vi "Autonomous Independent.vi"() -> ()   [LabVIEW 2016]
doc: "This VI is called when autonomous begins, and will automatically be terminated when autonomous ends. You can carry out timed or sensor driven robot movement independently without needing to return to the caller."
uses:
  <vilib>/Rock Robotics/WPI/Utilities/WPI_GetSetVariantRefNum.vi
  <vilib>/Rock Robotics/Network Tables/NT Read String.vi
  Robot Global Data.vi
  <vilib>/Rock Robotics/Network Tables/NT Write Numeric Array.vi
  <vilib>/Rock Robotics/WPI/RobotDrive/WPI_RobotDriveArcadeDrive_Standard(NoSaturation).vi
panel:
  out "Current Movement, for debugging":T1 {"Y Joystick Value" scale=1.0..-1.0; "X Joystick Value" scale=-1.0..1.0}
  in  "Array of robot movements":T2(array[cluster])=[{"X Joystick Value"=0.39393939393939403, "Y Joystick Value"=0.0, "Delay (sec)"=1.0, "Movement Name"="turn"}, {"X Joystick Value"=-0.3737373737373737, "Y Joystick Value"=0.0, "Delay (sec)"=1.0, "Movement Name"="turn back"}] {"Y Joystick Value" scale=1.0..-1.0; "X Joystick Value" scale=-1.0..1.0}
  # "Be sure to right-click and choose Data Operations>>Make Current Value default if you want to save the array values with the VI"
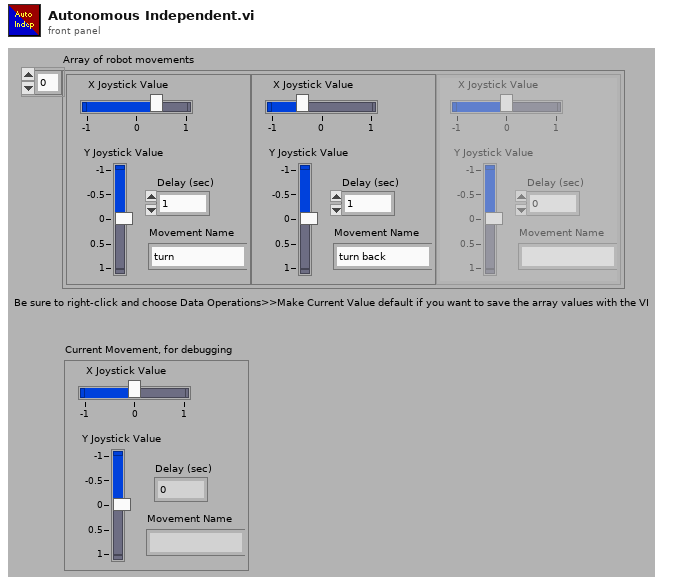
[diagram p1: front panel]
types:
  T1 = cluster{"X Joystick Value":dbl, "Y Joystick Value":dbl, "Delay (sec)":dbl, "Movement Name":string}
  T2 = cluster{"X Joystick Value":dbl, "Y Joystick Value":dbl, "Delay (sec)":dbl, "Movement Name":string}[]
  T3 = typedef "WPI_JoystickDevRef.ctl" = cluster{"Device":T4}
  T4 = typedef "WPI_JoystickDeviceEnum.ctl" = enum16{"USB 0", "USB 1", "USB 2", "USB 3", "USB 4", "USB 5"}
  T5 = typedef "WPI_RobotDriveDevRef.ctl" = cluster{"DevStatus":errorcluster, "Motors[]":T6[], "Square Inputs":bool, "Max Output":dbl}
  T6 = typedef "WPI_MotorControlDeviceRef.ctl" = cluster{"DeviceStatus":errorcluster, "Type":T7, "PWM":cluster{"PWM Channel":T8, "DeadBand":T9}, "CAN":cluster{"Device Number":u8, "SetOutput VI Ref":variant, "GetOutput VI Ref":variant, "Enable VI Ref":variant, "Disable VI Ref":variant, "Data":variant}, "Invert":bool}
  T7 = typedef "WPI_MotorControlType.ctl" = enum16{"PWM", "CAN"}
  T8 = typedef "FPGA_DIOPWMChannel.ctl" = enum8{"PWM 0", "PWM 1", "PWM 2", "PWM 3", "PWM 4", "PWM 5", "PWM 6", "PWM 7", "PWM 8", "PWM 9", "PWM MXP 0", "PWM MXP 1", "PWM MXP 2", "PWM MXP 3", "PWM MXP 4", "PWM MXP 5", "PWM MXP 6", "PWM MXP 7", "PWM MXP 8", "PWM MXP 9", "Invalid"}
  T9 = typedef "WPI_PWMDeadband.ctl" = cluster{"Name":string, "maxPositivePwm":i32, "minPositivePwm":i32, "centerPwm":i32, "maxNegativePwm":i32, "minNegativePwm":i32, "angularRange":u16}
  T10 = enum16{"Move Distance Setup", "Move to Distance", "Move End", "Place Gear Setup", "Place Gear Wait", "Place Gear End", "Angel Move Setup", "Angel Move Wait", "Angel Move End", "End Auto", "WaitForCompletion"}
  T11 = enum16{"Move Distance Setup", "Move to Distance", "Move End", "Place Gear Setup", "Place Gear Wait", "Place Gear End", "Angel Move Setup", "Angel Move Wait", "Angel Move End", "End Auto"}
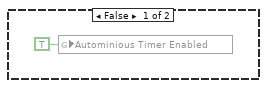
[diagram p6: hidden frame]
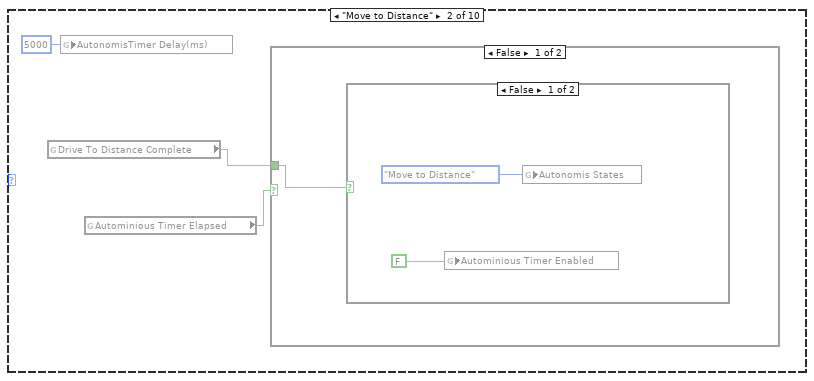
[diagram p7: hidden frame]
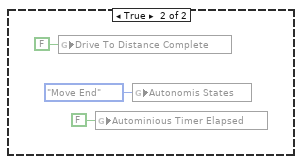
[diagram p8: hidden frame]
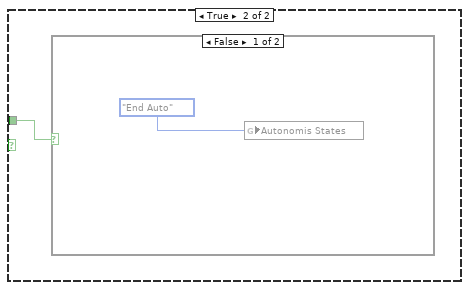
[diagram p9: hidden frame]
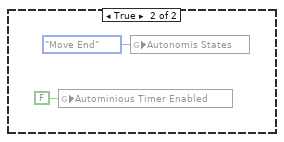
[diagram p10: hidden frame]
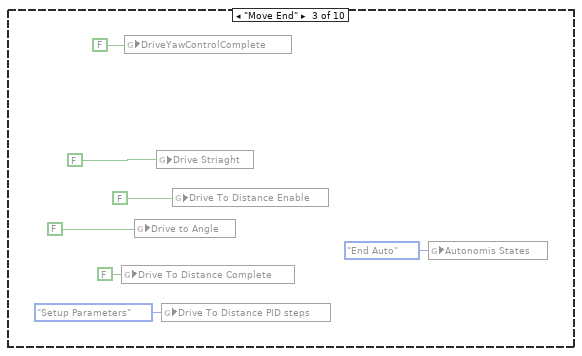
[diagram p11: hidden frame]
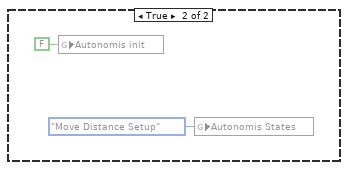
[diagram p19: hidden frame]
diagram:
  (unwired) "This function is run in parallel when the autonomous period begins. It will be terminated automatically when the period ends.\n\nNote that all Driver Station inputs are automatically latched and will not change once auto begins."
  # "initialize values for Move\nenable move to distnace  \nwait for ditance complete\nNext step"
  # "This tells you the autonomous selected\nfrom the dashboard"
  # "Every 20ms, report that we are running autonomous\ncode. Loop will abort the same time as the VI."
  # "This gives you the joystick value\nthat is often the throttle"
  # "This tells you the driver position\nand alliance color"
  n1 = while {
    stop <- FALSE stop-if-true
    n2 = call <vilib>:"WPI_DriverStationReport Robot Code State.vi"("Autonomous"=TRUE) -> ()  [unwired: 10 in, 1 out]
    n3 = Wait (ms)(milliseconds to wait=u32 20) -> ()  [unwired: 1 out]
  }
  n4 = call <vilib>:"WPI_DriverStationGet Alliance Info.vi"() -> ()  [unwired: 12 out]
  n5 = call <vilib>:"WPI_JoystickRefNum Registry Get.vi"("refnum name"="Joystick 0") -> ("JoystickDevRef"=w6:T3)  [unwired: 1 in, 9 out]
  n6 = call <vilib>:"WPI_JoystickGetValues.vi"("JoystickDevRef"=w6) -> ("Axes"=w3:dbl[])  [unwired: 6 in, 4 out]
  n7 = call-poly <vilib>:"NT Read Value.vi"("Name"="Auto Selector") -> ("String"=w1:string)  [unwired: 9 in, 1 out]
  n8 = call-poly <vilib>:"NT Write Value.vi"("Numeric Array"=w3, "Name"="Joystick 0/Axes") -> ()  [unwired: 9 in, 1 out]
  n9 = Index Array(array=w3, index=2) -> ()  [unwired: 1 out]
  n10 = disable-structure shown="Enabled" {
    disable-tunnel: w1 -> [w11 w42]
    frame Disabled {
      # "Use time and/or sensors to control how the robot drives."
      n11 = case shown="\"Alternative 1\"" w11 {
        frame Default {
          # "You can put your main auto here, or you can right-click on the case and make any\nother frame be the default case."
          # "This is the frame that will execute if no selection is made, or if it is not recognized"
        }
        frame "Alternative 1" {
          # "This sample code describes robot movements in an array. You can extend it to control other motors\non your robot. You can also use file I/O to move the data to a text file."
          n12 = call <vilib>:"WPI_RobotDriveRefNum Registry Get.vi"("refnum name"="Left and Right Motors") -> ("RobotDriveDevRef"=w13:T5)  [unwired: 1 in, 9 out]
          n13 = for {
            shift-right: [w21] -> _
            shift-left: w13 -> [w22]
            tunnel: "Array of robot movements" -> [w17] mode=indexing
            n14 = Unbundle By Name(w17) -> ("X Joystick Value"=w20:dbl, "Y Joystick Value"=w19:dbl, "Delay (sec)"=w18:dbl)  [unwired: 1 out]
            n15 = call-poly <vilib>:"WPI_RobotDriveArcadeDrive.vi"("Y axis value"=w19, "X axis value"=w20, "RobotDriveDevRef"=w22) -> ("Motor Values"=w15:dbl[], "RobotDriveDevRef"=w23:T5)  [unwired: 1 in, 6 out]
            n16 = call-poly <vilib>:"NT Write Value.vi"("Numeric Array"=w15, "Name"="RobotDrive Motors") -> ()  [unwired: 9 in, 1 out]
            n17 = call <vilib>:"WPI_RobotDriveDelayAndUpdateSafety.vi"("Delay (s)"=w18, "RobotDriveDevRef"=w23) -> ("RobotDriveDevRef 2"=w21:T5)  [unwired: 8 in, 1 out]
            "Current Movement, for debugging" <- w17
          }
        }
        frame "Alternative 2" {
          w25 = "RobotDrive Motors" ("Name")
          # "This is some simple sample code to drive your robot curving one direction and then the other."
          # "stand still"
          # "other way for 0.5 second"
          # "turn for 1 second"
          n18 = call <vilib>:"WPI_RobotDriveRefNum Registry Get.vi"("refnum name"="Left and Right Motors") -> ("RobotDriveDevRef"=w41:T5)  [unwired: 1 in, 9 out]
          n19 = call-poly <vilib>:"WPI_RobotDriveArcadeDrive.vi"("Y axis value"=0.5 ("X axis value"), "X axis value"=-0.25, "RobotDriveDevRef"=w41) -> ("Motor Values"=w24:dbl[], "RobotDriveDevRef"=w34:T5)  [unwired: 1 in, 6 out]
          n20 = call-poly <vilib>:"NT Write Value.vi"("Numeric Array"=w24, "Name"=w25) -> ()  [unwired: 9 in, 1 out]
          n21 = call <vilib>:"WPI_RobotDriveDelayAndUpdateSafety.vi"("Delay (s)"=1.0, "RobotDriveDevRef"=w34) -> ("RobotDriveDevRef 2"=w35:T5)  [unwired: 8 in, 1 out]
          n22 = call-poly <vilib>:"WPI_RobotDriveArcadeDrive.vi"("Y axis value"=-0.25 ("X axis value"), "X axis value"=0.5, "RobotDriveDevRef"=w35) -> ("Motor Values"=w26:dbl[], "RobotDriveDevRef"=w36:T5)  [unwired: 1 in, 6 out]
          n23 = call-poly <vilib>:"NT Write Value.vi"("Numeric Array"=w26, "Name"=w25) -> ()  [unwired: 9 in, 1 out]
          n24 = call <vilib>:"WPI_RobotDriveDelayAndUpdateSafety.vi"("Delay (s)"=0.5, "RobotDriveDevRef"=w36) -> ("RobotDriveDevRef 2"=w37:T5)  [unwired: 8 in, 1 out]
          n25 = call-poly <vilib>:"WPI_RobotDriveArcadeDrive.vi"("Y axis value"=0.0 ("X axis value"), "X axis value"=0.0, "RobotDriveDevRef"=w37) -> ("Motor Values"=w27:dbl[])  [unwired: 1 in, 7 out]
          n26 = call-poly <vilib>:"NT Write Value.vi"("Numeric Array"=w27, "Name"=w25) -> ()  [unwired: 9 in, 1 out]
        }
        frame "Your Turn" {
        }
      }
    }
    frame Enabled {
      n27 = case shown="\"Right\"" w42 {
        frame "False", Default {
        }
        frame "Do Nothing" {
        }
        frame "Drive Straight" {
          n28 = flat-sequence {
            frame #0 {
              n29 = global write "Robot Global Data.vi" "DriveYawControlComplete"(FALSE ("DriveYawControlRunning")) -> ()
              n30 = global write "Robot Global Data.vi" "Drive To Distance Complete"(FALSE ("Drive To Distance Complete")) -> ()
              n31 = global write "Robot Global Data.vi" "Drive Reset Encoders"(TRUE ("DriveYawControlRunning")) -> ()
              n32 = global write "Robot Global Data.vi" "Drive To Distance Enable"(FALSE ("Drive To Distance Enable")) -> ()
              n33 = global write "Robot Global Data.vi" "Drive to Angle"(FALSE ("Drive To Distance Enable")) -> ()
              n34 = global write "Robot Global Data.vi" "Drive To Distance PID steps"(enum16{"Setup Parameters", "Run PID", "Finish"}."Setup Parameters" ("Drive To Distance PID steps")) -> ()
              n35 = global write "Robot Global Data.vi" "Drive Striaght"(FALSE ("Drive To Distance Enable")) -> ()
              n36 = global write "Robot Global Data.vi" "Drive to Distance setpoint"(115.0 ("Drive to Distance setpoint")) -> ()
              n37 = global write "Robot Global Data.vi" "Nav Reset Yaw"(TRUE ("Drive To Distance Enable")) -> ()
              n38 = Wait (ms)(milliseconds to wait=u32 200) -> ()  [unwired: 1 out]
            }
            frame #1 {
              n39 = global write "Robot Global Data.vi" "Drive To Distance Enable"(TRUE ("Drive To Distance Enable")) -> ()
            }
            frame #2 {
              n40 = while {
                stop <- w55 stop-if-true
                n41 = global read "Robot Global Data.vi" "Drive To Distance Complete"() -> (w55:bool)
                n42 = Wait (ms)(milliseconds to wait=u32 10) -> ()  [unwired: 1 out]
              }
              n43 = global write "Robot Global Data.vi" "Drive Reset Encoders"(FALSE ("DriveYawControlRunning")) -> ()
            }
            frame #3 {
              n44 = global write "Robot Global Data.vi" "Drive To Distance Complete"(FALSE ("Drive To Distance Complete")) -> ()
              n45 = global write "Robot Global Data.vi" "DriveYawControlComplete"(FALSE ("DriveYawControlRunning")) -> ()
              n46 = global write "Robot Global Data.vi" "Drive to Angle"(FALSE ("Drive To Distance Enable")) -> ()
              n47 = global write "Robot Global Data.vi" "Drive Striaght"(FALSE ("Drive To Distance Enable")) -> ()
              n48 = global write "Robot Global Data.vi" "Drive To Distance PID steps"(enum16{"Setup Parameters", "Run PID", "Finish"}."Setup Parameters" ("Drive To Distance PID steps")) -> ()
              n49 = global write "Robot Global Data.vi" "Drive To Distance Enable"(FALSE ("Drive To Distance Enable")) -> ()
            }
            frame #4 {
            }
            frame #5 {
            }
          }
        }
        frame "Left" {
          n50 = flat-sequence {
            frame #0 {
              n51 = global write "Robot Global Data.vi" "DriveYawControlComplete"(FALSE ("DriveYawControlRunning")) -> ()
              n52 = global write "Robot Global Data.vi" "Drive To Distance Complete"(FALSE ("Drive To Distance Complete")) -> ()
              n53 = global write "Robot Global Data.vi" "Drive Reset Encoders"(TRUE ("DriveYawControlRunning")) -> ()
              n54 = global write "Robot Global Data.vi" "Drive To Distance Enable"(FALSE ("Drive To Distance Enable")) -> ()
              n55 = global write "Robot Global Data.vi" "Drive to Angle"(FALSE ("Drive To Distance Enable")) -> ()
              n56 = global write "Robot Global Data.vi" "Drive To Distance PID steps"(enum16{"Setup Parameters", "Run PID", "Finish"}."Setup Parameters" ("Drive To Distance PID steps")) -> ()
              n57 = global write "Robot Global Data.vi" "Drive Striaght"(FALSE ("Drive To Distance Enable")) -> ()
              n58 = global write "Robot Global Data.vi" "Drive to Distance setpoint"(150.0 ("Drive to Distance setpoint")) -> ()
              n59 = global write "Robot Global Data.vi" "Nav Reset Yaw"(TRUE ("Drive To Distance Enable")) -> ()
              n60 = global write "Robot Global Data.vi" "Drive to Distance Direction"(enum16{"Y direction", "X Direction"}."Y direction" ("Drive to Distance Direction")) -> ()
              n61 = Wait (ms)(milliseconds to wait=u32 200) -> ()  [unwired: 1 out]
            }
            frame #1 {
              n62 = global write "Robot Global Data.vi" "Drive To Distance Enable"(TRUE ("Drive To Distance Enable")) -> ()
            }
            frame #2 {
              n63 = while {
                stop <- w76 stop-if-true
                n64 = global read "Robot Global Data.vi" "Drive To Distance Complete"() -> (w76:bool)
                n65 = Wait (ms)(milliseconds to wait=u32 10) -> ()  [unwired: 1 out]
              }
              n66 = global write "Robot Global Data.vi" "Drive Reset Encoders"(FALSE ("DriveYawControlRunning")) -> ()
            }
            frame #3 {
              n67 = global write "Robot Global Data.vi" "Drive To Distance Complete"(FALSE ("Drive To Distance Complete")) -> ()
              n68 = global write "Robot Global Data.vi" "DriveYawControlComplete"(FALSE ("DriveYawControlRunning")) -> ()
              n69 = global write "Robot Global Data.vi" "Drive to Angle"(FALSE ("Drive To Distance Enable")) -> ()
              n70 = global write "Robot Global Data.vi" "Drive Striaght"(FALSE ("Drive To Distance Enable")) -> ()
              n71 = global write "Robot Global Data.vi" "Drive To Distance PID steps"(enum16{"Setup Parameters", "Run PID", "Finish"}."Setup Parameters" ("Drive To Distance PID steps")) -> ()
              n72 = global write "Robot Global Data.vi" "Drive To Distance Enable"(FALSE ("Drive To Distance Enable")) -> ()
            }
            frame #4 {
              n73 = global write "Robot Global Data.vi" "Drive Reset Encoders"(TRUE ("DriveYawControlRunning")) -> ()
              n74 = global write "Robot Global Data.vi" "GearPlace"(TRUE ("GearPlace")) -> ()
            }
            frame #5 {
              n75 = while {
                stop <- w87 stop-if-true
                n76 = global read "Robot Global Data.vi" "GearPlaceComplete"() -> (w87:bool)
                n77 = Wait (ms)(milliseconds to wait=u32 50) -> ()  [unwired: 1 out]
              }
            }
            frame #6 {
              n78 = global write "Robot Global Data.vi" "DriveYawControlComplete"(FALSE ("DriveYawControlRunning")) -> ()
              n79 = global write "Robot Global Data.vi" "Drive To Distance Complete"(FALSE ("Drive To Distance Complete")) -> ()
              n80 = global write "Robot Global Data.vi" "Drive Reset Encoders"(TRUE ("DriveYawControlRunning")) -> ()
              n81 = global write "Robot Global Data.vi" "Drive To Distance Enable"(FALSE ("Drive To Distance Enable")) -> ()
              n82 = global write "Robot Global Data.vi" "Drive to Angle"(FALSE ("Drive To Distance Enable")) -> ()
              n83 = global write "Robot Global Data.vi" "Drive To Distance PID steps"(enum16{"Setup Parameters", "Run PID", "Finish"}."Setup Parameters" ("Drive To Distance PID steps")) -> ()
              n84 = global write "Robot Global Data.vi" "Drive Striaght"(FALSE ("Drive To Distance Enable")) -> ()
              n85 = global write "Robot Global Data.vi" "Drive to Distance Direction"(enum16{"Y direction", "X Direction"}."Y direction" ("Drive to Distance Direction")) -> ()
              n86 = global write "Robot Global Data.vi" "Drive to Distance setpoint"(-12.0 ("Drive to Distance setpoint")) -> ()
              n87 = global write "Robot Global Data.vi" "GearPlace"(FALSE ("GearPlace")) -> ()
              n88 = global write "Robot Global Data.vi" "Nav Reset Yaw"(TRUE ("Drive To Distance Enable")) -> ()
              n89 = Wait (ms)(milliseconds to wait=u32 200) -> ()  [unwired: 1 out]
            }
            frame #7 {
              n90 = global write "Robot Global Data.vi" "Drive To Distance Enable"(TRUE ("Drive To Distance Enable")) -> ()
            }
            frame #8 {
              n91 = while {
                stop <- w102 stop-if-true
                n92 = global read "Robot Global Data.vi" "Drive To Distance Complete"() -> (w102:bool)
                n93 = Wait (ms)(milliseconds to wait=u32 50) -> ()  [unwired: 1 out]
              }
              n94 = global write "Robot Global Data.vi" "Drive Reset Encoders"(FALSE ("DriveYawControlRunning")) -> ()
            }
            frame #9 {
              n95 = global write "Robot Global Data.vi" "Drive To Distance Complete"(FALSE ("Drive To Distance Complete")) -> ()
              n96 = global write "Robot Global Data.vi" "DriveYawControlComplete"(FALSE ("DriveYawControlRunning")) -> ()
              n97 = global write "Robot Global Data.vi" "Drive to Angle"(FALSE ("Drive To Distance Enable")) -> ()
              n98 = global write "Robot Global Data.vi" "Drive Striaght"(FALSE ("Drive To Distance Enable")) -> ()
              n99 = global write "Robot Global Data.vi" "Drive To Distance PID steps"(enum16{"Setup Parameters", "Run PID", "Finish"}."Setup Parameters" ("Drive To Distance PID steps")) -> ()
              n100 = global write "Robot Global Data.vi" "Drive To Distance Enable"(FALSE ("Drive To Distance Enable")) -> ()
            }
            frame #10 {
              n101 = global write "Robot Global Data.vi" "GearPlace"(FALSE ("GearPlace")) -> ()
            }
            frame #11 {
              n102 = disable-structure shown="Disabled" {
                frame Disabled {
                  n103 = global write "Robot Global Data.vi" "DriveYawControlComplete"(FALSE ("DriveYawControlRunning")) -> ()
                  n104 = global write "Robot Global Data.vi" "Drive To Distance Complete"(FALSE ("Drive To Distance Complete")) -> ()
                  n105 = global write "Robot Global Data.vi" "Drive Reset Encoders"(TRUE ("DriveYawControlRunning")) -> ()
                  n106 = global write "Robot Global Data.vi" "Drive To Distance Enable"(FALSE ("Drive To Distance Enable")) -> ()
                  n107 = global write "Robot Global Data.vi" "Drive to Angle"(FALSE ("Drive To Distance Enable")) -> ()
                  n108 = global write "Robot Global Data.vi" "Drive To Distance PID steps"(enum16{"Setup Parameters", "Run PID", "Finish"}."Setup Parameters" ("Drive To Distance PID steps")) -> ()
                  n109 = global write "Robot Global Data.vi" "Drive Striaght"(FALSE ("Drive To Distance Enable")) -> ()
                  n110 = global write "Robot Global Data.vi" "Drive to Distance setpoint"(24.0 ("Drive to Distance setpoint")) -> ()
                  n111 = global write "Robot Global Data.vi" "Gear Holder Open"(FALSE ("Gear Holder Open")) -> ()
                  n112 = global write "Robot Global Data.vi" "Nav Reset Yaw"(TRUE ("Drive To Distance Enable")) -> ()
                  n113 = global write "Robot Global Data.vi" "Drive to Distance Direction"(enum16{"Y direction", "X Direction"}."X Direction" ("Drive to Distance Direction")) -> ()
                  n114 = Wait (ms)(milliseconds to wait=u32 200) -> ()  [unwired: 1 out]
                }
                frame Enabled {
                }
              }
            }
            frame #12 {
              n115 = disable-structure shown="Disabled" {
                frame Disabled {
                  n116 = global write "Robot Global Data.vi" "Drive To Distance Enable"(TRUE ("Drive To Distance Enable")) -> ()
                }
                frame Enabled {
                }
              }
            }
            frame #13 {
              n117 = disable-structure shown="Disabled" {
                frame Disabled {
                  n118 = while {
                    stop <- w125 stop-if-true
                    n119 = global read "Robot Global Data.vi" "Drive To Distance Complete"() -> (w125:bool)
                    n120 = Wait (ms)(milliseconds to wait=u32 10) -> ()  [unwired: 1 out]
                  }
                  n121 = global write "Robot Global Data.vi" "Drive Reset Encoders"(FALSE ("DriveYawControlRunning")) -> ()
                }
                frame Enabled {
                }
              }
            }
            frame #14 {
              n122 = disable-structure shown="Disabled" {
                frame Disabled {
                  n123 = global write "Robot Global Data.vi" "Drive To Distance Complete"(FALSE ("Drive To Distance Complete")) -> ()
                  n124 = global write "Robot Global Data.vi" "DriveYawControlComplete"(FALSE ("DriveYawControlRunning")) -> ()
                  n125 = global write "Robot Global Data.vi" "Drive to Angle"(FALSE ("Drive To Distance Enable")) -> ()
                  n126 = global write "Robot Global Data.vi" "Drive Striaght"(FALSE ("Drive To Distance Enable")) -> ()
                  n127 = global write "Robot Global Data.vi" "Drive To Distance PID steps"(enum16{"Setup Parameters", "Run PID", "Finish"}."Setup Parameters" ("Drive To Distance PID steps")) -> ()
                  n128 = global write "Robot Global Data.vi" "Drive To Distance Enable"(FALSE ("Drive To Distance Enable")) -> ()
                }
                frame Enabled {
                }
              }
            }
          }
        }
        frame "Center" {
          n129 = flat-sequence {
            frame #0 {
              n130 = global write "Robot Global Data.vi" "DriveYawControlComplete"(FALSE ("DriveYawControlRunning")) -> ()
              n131 = global write "Robot Global Data.vi" "Drive To Distance Complete"(FALSE ("Drive To Distance Complete")) -> ()
              n132 = global write "Robot Global Data.vi" "Drive Reset Encoders"(TRUE ("DriveYawControlRunning")) -> ()
              n133 = global write "Robot Global Data.vi" "Drive To Distance Enable"(FALSE ("Drive To Distance Enable")) -> ()
              n134 = global write "Robot Global Data.vi" "Drive to Angle"(FALSE ("Drive To Distance Enable")) -> ()
              n135 = global write "Robot Global Data.vi" "Drive To Distance PID steps"(enum16{"Setup Parameters", "Run PID", "Finish"}."Setup Parameters" ("Drive To Distance PID steps")) -> ()
              n136 = global write "Robot Global Data.vi" "Drive Striaght"(FALSE ("Drive To Distance Enable")) -> ()
              n137 = global write "Robot Global Data.vi" "Drive to Distance setpoint"(100.0 ("Drive to Distance setpoint")) -> ()
              n138 = global write "Robot Global Data.vi" "Nav Reset Yaw"(TRUE ("Drive To Distance Enable")) -> ()
              n139 = global write "Robot Global Data.vi" "Drive to Distance Direction"(enum16{"Y direction", "X Direction"}."Y direction" ("Drive to Distance Direction")) -> ()
              n140 = Wait (ms)(milliseconds to wait=u32 400) -> ()  [unwired: 1 out]
            }
            frame #1 {
              n141 = global write "Robot Global Data.vi" "Drive To Distance Enable"(TRUE ("Drive To Distance Enable")) -> ()
            }
            frame #2 {
              n142 = while {
                stop <- w146 stop-if-true
                n143 = global read "Robot Global Data.vi" "Drive To Distance Complete"() -> (w146:bool)
                n144 = Wait (ms)(milliseconds to wait=u32 10) -> ()  [unwired: 1 out]
              }
              n145 = global write "Robot Global Data.vi" "Drive Reset Encoders"(FALSE ("DriveYawControlRunning")) -> ()
            }
            frame #3 {
              n146 = global write "Robot Global Data.vi" "Drive To Distance Complete"(FALSE ("Drive To Distance Complete")) -> ()
              n147 = global write "Robot Global Data.vi" "DriveYawControlComplete"(FALSE ("DriveYawControlRunning")) -> ()
              n148 = global write "Robot Global Data.vi" "Drive to Angle"(FALSE ("Drive To Distance Enable")) -> ()
              n149 = global write "Robot Global Data.vi" "Drive Striaght"(FALSE ("Drive To Distance Enable")) -> ()
              n150 = global write "Robot Global Data.vi" "Drive To Distance PID steps"(enum16{"Setup Parameters", "Run PID", "Finish"}."Setup Parameters" ("Drive To Distance PID steps")) -> ()
              n151 = global write "Robot Global Data.vi" "Drive To Distance Enable"(FALSE ("Drive To Distance Enable")) -> ()
            }
            frame #4 {
              n152 = global write "Robot Global Data.vi" "Drive Reset Encoders"(TRUE ("DriveYawControlRunning")) -> ()
              n153 = global write "Robot Global Data.vi" "GearPlace"(TRUE ("GearPlace")) -> ()
              n154 = Wait (ms)(milliseconds to wait=u32 10) -> ()  [unwired: 1 out]
            }
            frame #5 {
              n155 = while {
                stop <- w157 stop-if-true
                n156 = global read "Robot Global Data.vi" "GearPlaceComplete"() -> (w157:bool)
                n157 = Wait (ms)(milliseconds to wait=u32 50) -> ()  [unwired: 1 out]
              }
            }
            frame #6 {
              n158 = global write "Robot Global Data.vi" "DriveYawControlComplete"(FALSE ("DriveYawControlRunning")) -> ()
              n159 = global write "Robot Global Data.vi" "Drive To Distance Complete"(FALSE ("Drive To Distance Complete")) -> ()
              n160 = global write "Robot Global Data.vi" "Drive Reset Encoders"(TRUE ("DriveYawControlRunning")) -> ()
              n161 = global write "Robot Global Data.vi" "Drive To Distance Enable"(FALSE ("Drive To Distance Enable")) -> ()
              n162 = global write "Robot Global Data.vi" "Drive to Angle"(FALSE ("Drive To Distance Enable")) -> ()
              n163 = global write "Robot Global Data.vi" "Drive To Distance PID steps"(enum16{"Setup Parameters", "Run PID", "Finish"}."Setup Parameters" ("Drive To Distance PID steps")) -> ()
              n164 = global write "Robot Global Data.vi" "Drive Striaght"(FALSE ("Drive To Distance Enable")) -> ()
              n165 = global write "Robot Global Data.vi" "Drive to Distance Direction"(enum16{"Y direction", "X Direction"}."Y direction" ("Drive to Distance Direction")) -> ()
              n166 = global write "Robot Global Data.vi" "Drive to Distance setpoint"(-12.0 ("Drive to Distance setpoint")) -> ()
              n167 = global write "Robot Global Data.vi" "Nav Reset Yaw"(TRUE ("Drive To Distance Enable")) -> ()
              n168 = global write "Robot Global Data.vi" "GearPlace"(FALSE ("GearPlace")) -> ()
              n169 = Wait (ms)(milliseconds to wait=u32 200) -> ()  [unwired: 1 out]
            }
            frame #7 {
              n170 = global write "Robot Global Data.vi" "Drive To Distance Enable"(TRUE ("Drive To Distance Enable")) -> ()
            }
            frame #8 {
              n171 = while {
                stop <- w173 stop-if-true
                n172 = global read "Robot Global Data.vi" "Drive To Distance Complete"() -> (w173:bool)
                n173 = Wait (ms)(milliseconds to wait=u32 50) -> ()  [unwired: 1 out]
              }
              n174 = global write "Robot Global Data.vi" "Drive Reset Encoders"(FALSE ("DriveYawControlRunning")) -> ()
            }
            frame #9 {
              n175 = global write "Robot Global Data.vi" "Drive To Distance Complete"(FALSE ("Drive To Distance Complete")) -> ()
              n176 = global write "Robot Global Data.vi" "DriveYawControlComplete"(FALSE ("DriveYawControlRunning")) -> ()
              n177 = global write "Robot Global Data.vi" "Drive to Angle"(FALSE ("Drive To Distance Enable")) -> ()
              n178 = global write "Robot Global Data.vi" "Drive Striaght"(FALSE ("Drive To Distance Enable")) -> ()
              n179 = global write "Robot Global Data.vi" "Drive To Distance PID steps"(enum16{"Setup Parameters", "Run PID", "Finish"}."Setup Parameters" ("Drive To Distance PID steps")) -> ()
              n180 = global write "Robot Global Data.vi" "Drive To Distance Enable"(FALSE ("Drive To Distance Enable")) -> ()
            }
          }
        }
        frame "Right" {
          n181 = flat-sequence {
            frame #0 {
              n182 = global write "Robot Global Data.vi" "DriveYawControlComplete"(FALSE ("DriveYawControlRunning")) -> ()
              n183 = global write "Robot Global Data.vi" "Drive To Distance Complete"(FALSE ("Drive To Distance Complete")) -> ()
              n184 = global write "Robot Global Data.vi" "Drive Reset Encoders"(TRUE ("DriveYawControlRunning")) -> ()
              n185 = global write "Robot Global Data.vi" "Drive To Distance Enable"(FALSE ("Drive To Distance Enable")) -> ()
              n186 = global write "Robot Global Data.vi" "Drive to Angle"(FALSE ("Drive To Distance Enable")) -> ()
              n187 = global write "Robot Global Data.vi" "Drive To Distance PID steps"(enum16{"Setup Parameters", "Run PID", "Finish"}."Setup Parameters" ("Drive To Distance PID steps")) -> ()
              n188 = global write "Robot Global Data.vi" "Drive Striaght"(FALSE ("Drive To Distance Enable")) -> ()
              n189 = global write "Robot Global Data.vi" "Drive to Distance setpoint"(150.0 ("Drive to Distance setpoint")) -> ()
              n190 = global write "Robot Global Data.vi" "Nav Reset Yaw"(TRUE ("Drive To Distance Enable")) -> ()
              n191 = global write "Robot Global Data.vi" "Drive to Distance Direction"(enum16{"Y direction", "X Direction"}."Y direction" ("Drive to Distance Direction")) -> ()
              n192 = Wait (ms)(milliseconds to wait=u32 400) -> ()  [unwired: 1 out]
            }
            frame #1 {
              n193 = global write "Robot Global Data.vi" "Drive To Distance Enable"(TRUE ("Drive To Distance Enable")) -> ()
            }
            frame #2 {
              n194 = while {
                stop <- w194 stop-if-true
                n195 = global read "Robot Global Data.vi" "Drive To Distance Complete"() -> (w194:bool)
                n196 = Wait (ms)(milliseconds to wait=u32 50) -> ()  [unwired: 1 out]
              }
              n197 = global write "Robot Global Data.vi" "Drive Reset Encoders"(FALSE ("DriveYawControlRunning")) -> ()
            }
            frame #3 {
              n198 = global write "Robot Global Data.vi" "Drive To Distance Complete"(FALSE ("Drive To Distance Complete")) -> ()
              n199 = global write "Robot Global Data.vi" "DriveYawControlComplete"(FALSE ("DriveYawControlRunning")) -> ()
              n200 = global write "Robot Global Data.vi" "Drive to Angle"(FALSE ("Drive To Distance Enable")) -> ()
              n201 = global write "Robot Global Data.vi" "Drive Striaght"(FALSE ("Drive To Distance Enable")) -> ()
              n202 = global write "Robot Global Data.vi" "Drive To Distance PID steps"(enum16{"Setup Parameters", "Run PID", "Finish"}."Setup Parameters" ("Drive To Distance PID steps")) -> ()
              n203 = global write "Robot Global Data.vi" "Drive To Distance Enable"(FALSE ("Drive To Distance Enable")) -> ()
            }
            frame #4 {
              n204 = global write "Robot Global Data.vi" "Drive Reset Encoders"(TRUE ("DriveYawControlRunning")) -> ()
              n205 = global write "Robot Global Data.vi" "GearPlace"(TRUE ("GearPlace")) -> ()
            }
            frame #5 {
              n206 = while {
                stop <- w205 stop-if-true
                n207 = global read "Robot Global Data.vi" "GearPlaseTimerElapsed"() -> (w205:bool)
                n208 = Wait (ms)(milliseconds to wait=u32 50) -> ()  [unwired: 1 out]
              }
            }
            frame #6 {
              n209 = global write "Robot Global Data.vi" "DriveYawControlComplete"(FALSE ("DriveYawControlRunning")) -> ()
              n210 = global write "Robot Global Data.vi" "Drive To Distance Complete"(FALSE ("Drive To Distance Complete")) -> ()
              n211 = global write "Robot Global Data.vi" "Drive Reset Encoders"(TRUE ("DriveYawControlRunning")) -> ()
              n212 = global write "Robot Global Data.vi" "Drive To Distance Enable"(FALSE ("Drive To Distance Enable")) -> ()
              n213 = global write "Robot Global Data.vi" "Drive to Angle"(FALSE ("Drive To Distance Enable")) -> ()
              n214 = global write "Robot Global Data.vi" "Drive To Distance PID steps"(enum16{"Setup Parameters", "Run PID", "Finish"}."Setup Parameters" ("Drive To Distance PID steps")) -> ()
              n215 = global write "Robot Global Data.vi" "Drive Striaght"(FALSE ("Drive To Distance Enable")) -> ()
              n216 = global write "Robot Global Data.vi" "Drive to Distance Direction"(enum16{"Y direction", "X Direction"}."Y direction" ("Drive to Distance Direction")) -> ()
              n217 = global write "Robot Global Data.vi" "Drive to Distance setpoint"(-12.0 ("Drive to Distance setpoint")) -> ()
              n218 = global write "Robot Global Data.vi" "GearPlace"(FALSE ("GearPlace")) -> ()
              n219 = global write "Robot Global Data.vi" "Nav Reset Yaw"(TRUE ("Drive To Distance Enable")) -> ()
              n220 = Wait (ms)(milliseconds to wait=u32 200) -> ()  [unwired: 1 out]
            }
            frame #7 {
              n221 = global write "Robot Global Data.vi" "Drive To Distance Enable"(TRUE ("Drive To Distance Enable")) -> ()
            }
            frame #8 {
              n222 = while {
                stop <- w221 stop-if-true
                n223 = global read "Robot Global Data.vi" "Drive To Distance Complete"() -> (w221:bool)
                n224 = Wait (ms)(milliseconds to wait=u32 50) -> ()  [unwired: 1 out]
              }
              n225 = global write "Robot Global Data.vi" "Drive Reset Encoders"(FALSE ("DriveYawControlRunning")) -> ()
            }
            frame #9 {
              n226 = global write "Robot Global Data.vi" "Drive To Distance Complete"(FALSE ("Drive To Distance Complete")) -> ()
              n227 = global write "Robot Global Data.vi" "DriveYawControlComplete"(FALSE ("DriveYawControlRunning")) -> ()
              n228 = global write "Robot Global Data.vi" "Drive to Angle"(FALSE ("Drive To Distance Enable")) -> ()
              n229 = global write "Robot Global Data.vi" "Drive Striaght"(FALSE ("Drive To Distance Enable")) -> ()
              n230 = global write "Robot Global Data.vi" "Drive To Distance PID steps"(enum16{"Setup Parameters", "Run PID", "Finish"}."Setup Parameters" ("Drive To Distance PID steps")) -> ()
              n231 = global write "Robot Global Data.vi" "Drive To Distance Enable"(FALSE ("Drive To Distance Enable")) -> ()
            }
            frame #10 {
              n232 = disable-structure shown="Disabled" {
                frame Disabled {
                  n233 = global write "Robot Global Data.vi" "DriveYawControlComplete"(FALSE ("DriveYawControlRunning")) -> ()
                  n234 = global write "Robot Global Data.vi" "Drive To Distance Complete"(FALSE ("Drive To Distance Complete")) -> ()
                  n235 = global write "Robot Global Data.vi" "Drive Reset Encoders"(TRUE ("DriveYawControlRunning")) -> ()
                  n236 = global write "Robot Global Data.vi" "Drive To Distance Enable"(FALSE ("Drive To Distance Enable")) -> ()
                  n237 = global write "Robot Global Data.vi" "Drive to Angle"(FALSE ("Drive To Distance Enable")) -> ()
                  n238 = global write "Robot Global Data.vi" "Drive To Distance PID steps"(enum16{"Setup Parameters", "Run PID", "Finish"}."Setup Parameters" ("Drive To Distance PID steps")) -> ()
                  n239 = global write "Robot Global Data.vi" "Drive Striaght"(FALSE ("Drive To Distance Enable")) -> ()
                  n240 = global write "Robot Global Data.vi" "Drive to Distance setpoint"(-24.0 ("Drive to Distance setpoint")) -> ()
                  n241 = global write "Robot Global Data.vi" "Gear Holder Open"(FALSE ("Gear Holder Open")) -> ()
                  n242 = global write "Robot Global Data.vi" "Nav Reset Yaw"(TRUE ("Drive To Distance Enable")) -> ()
                  n243 = global write "Robot Global Data.vi" "Drive to Distance Direction"(enum16{"Y direction", "X Direction"}."X Direction" ("Drive to Distance Direction")) -> ()
                  n244 = Wait (ms)(milliseconds to wait=u32 200) -> ()  [unwired: 1 out]
                }
                frame Enabled {
                }
              }
            }
            frame #11 {
              n245 = disable-structure shown="Disabled" {
                frame Disabled {
                  n246 = global write "Robot Global Data.vi" "Drive To Distance Enable"(TRUE ("Drive To Distance Enable")) -> ()
                }
                frame Enabled {
                }
              }
            }
            frame #12 {
              n247 = disable-structure shown="Disabled" {
                frame Disabled {
                  n248 = while {
                    stop <- w242 stop-if-true
                    n249 = global read "Robot Global Data.vi" "Drive To Distance Complete"() -> (w242:bool)
                    n250 = Wait (ms)(milliseconds to wait=u32 10) -> ()  [unwired: 1 out]
                  }
                  n251 = global write "Robot Global Data.vi" "Drive Reset Encoders"(FALSE ("DriveYawControlRunning")) -> ()
                }
                frame Enabled {
                }
              }
            }
            frame #13 {
              n252 = disable-structure shown="Disabled" {
                frame Disabled {
                  n253 = global write "Robot Global Data.vi" "Drive To Distance Complete"(FALSE ("Drive To Distance Complete")) -> ()
                  n254 = global write "Robot Global Data.vi" "DriveYawControlComplete"(FALSE ("DriveYawControlRunning")) -> ()
                  n255 = global write "Robot Global Data.vi" "Drive to Angle"(FALSE ("Drive To Distance Enable")) -> ()
                  n256 = global write "Robot Global Data.vi" "Drive Striaght"(FALSE ("Drive To Distance Enable")) -> ()
                  n257 = global write "Robot Global Data.vi" "Drive To Distance PID steps"(enum16{"Setup Parameters", "Run PID", "Finish"}."Setup Parameters" ("Drive To Distance PID steps")) -> ()
                  n258 = global write "Robot Global Data.vi" "Drive to Distance Direction"(enum16{"Y direction", "X Direction"}."Y direction" ("Drive to Distance Direction")) -> ()
                  n259 = global write "Robot Global Data.vi" "Drive To Distance Enable"(FALSE ("Drive To Distance Enable")) -> ()
                }
                frame Enabled {
                }
              }
            }
          }
        }
      }
    }
  }
  n260 = disable-structure shown="Disabled" {
    disable-tunnel: w1 -> [w251 _]
    frame Disabled {
      n261 = case shown="\"Right\"" w251 {
        frame "Do Nothing", Default {
        }
        frame "Center" {
        }
        frame "Drive Straight" {
        }
        frame "Left" {
        }
        frame "Right" {
          n262 = global read "Robot Global Data.vi" "Autonomis init"() -> (w252:bool)
          n263 = case shown="False" w252 {
            frame False {
              n264 = global read "Robot Global Data.vi" "Autonomis States"() -> (w253:T10)
              n265 = case shown="\"Move Distance Setup\", Default" w253 {
                frame "Move Distance Setup", Default {
                  n266 = global write "Robot Global Data.vi" "DriveYawControlComplete"(FALSE ("DriveYawControlRunning")) -> ()
                  n267 = global write "Robot Global Data.vi" "Drive To Distance Complete"(FALSE ("Drive To Distance Complete")) -> ()
                  n268 = global write "Robot Global Data.vi" "Drive Reset Encoders"(TRUE ("DriveYawControlRunning")) -> ()
                  n269 = global write "Robot Global Data.vi" "Drive To Distance Enable"(FALSE ("Drive To Distance Enable")) -> ()
                  n270 = global write "Robot Global Data.vi" "Drive to Angle"(FALSE ("Drive To Distance Enable")) -> ()
                  n271 = global write "Robot Global Data.vi" "Drive Striaght"(FALSE ("Drive To Distance Enable")) -> ()
                  n272 = global write "Robot Global Data.vi" "Nav Reset Yaw"(TRUE ("Drive To Distance Enable")) -> ()
                  n273 = global write "Robot Global Data.vi" "Drive to Distance setpoint"(115.0 ("Drive to Distance setpoint")) -> ()
                  n274 = global read "Robot Global Data.vi" "Autominious Timer Elapsed"() -> (w255:bool)
                  n275 = global write "Robot Global Data.vi" "AutonomisTimer Delay(ms)"(u32 200 ("AutonomisTimer Delay(ms)")) -> ()
                  n276 = case shown="True" w255 {
                    frame False {
                      n277 = global write "Robot Global Data.vi" "Autominious Timer Enabled"(TRUE ("Autominious Timer Enabled")) -> ()
                    }
                    frame True {
                      n278 = global write "Robot Global Data.vi" "Drive To Distance Enable"(FALSE ("Drive To Distance Enable")) -> ()
                      n279 = global write "Robot Global Data.vi" "Drive Reset Encoders"(FALSE ("DriveYawControlRunning")) -> ()
                      n280 = global write "Robot Global Data.vi" "Autominious Timer Enabled"(FALSE ("Autominious Timer Enabled")) -> ()
                      n281 = global write "Robot Global Data.vi" "Autonomis States"(T10."Move to Distance" ("Autonomis States")) -> ()
                    }
                  }
                }
                frame "Move to Distance" {
                  n282 = global read "Robot Global Data.vi" "Drive To Distance Complete"() -> (w271:bool)
                  n283 = global write "Robot Global Data.vi" "AutonomisTimer Delay(ms)"(u32 5000 ("AutonomisTimer Delay(ms)")) -> ()
                  n284 = global read "Robot Global Data.vi" "Autominious Timer Elapsed"() -> (w269:bool)
                  n285 = case shown="False" w269 {
                    tunnel: w271 -> [w272 w278]
                    frame False {
                      n286 = case shown="False" w272 {
                        frame False {
                          n287 = global write "Robot Global Data.vi" "Autominious Timer Enabled"(FALSE ("Autominious Timer Enabled")) -> ()
                          n288 = global write "Robot Global Data.vi" "Autonomis States"(T10."Move to Distance" ("Autonomis States")) -> ()
                        }
                        frame True {
                          n289 = global write "Robot Global Data.vi" "Drive To Distance Complete"(FALSE ("Drive To Distance Complete")) -> ()
                          n290 = global write "Robot Global Data.vi" "Autominious Timer Elapsed"(FALSE ("Autominious Timer Elapsed")) -> ()
                          n291 = global write "Robot Global Data.vi" "Autonomis States"(T10."Move End" ("Autonomis States")) -> ()
                        }
                      }
                    }
                    frame True {
                      n292 = case shown="False" w278 {
                        frame False {
                          n293 = global write "Robot Global Data.vi" "Autonomis States"(T10."End Auto" ("Autonomis States")) -> ()
                        }
                        frame True {
                          n294 = global write "Robot Global Data.vi" "Autominious Timer Enabled"(FALSE ("Autominious Timer Enabled")) -> ()
                          n295 = global write "Robot Global Data.vi" "Autonomis States"(T10."Move End" ("Autonomis States")) -> ()
                        }
                      }
                    }
                  }
                }
                frame "Move End" {
                  n296 = global write "Robot Global Data.vi" "Drive To Distance Complete"(FALSE ("Drive To Distance Complete")) -> ()
                  n297 = global write "Robot Global Data.vi" "DriveYawControlComplete"(FALSE ("DriveYawControlRunning")) -> ()
                  n298 = global write "Robot Global Data.vi" "Drive to Angle"(FALSE ("Drive To Distance Enable")) -> ()
                  n299 = global write "Robot Global Data.vi" "Drive Striaght"(FALSE ("Drive To Distance Enable")) -> ()
                  n300 = global write "Robot Global Data.vi" "Drive To Distance PID steps"(enum16{"Setup Parameters", "Run PID", "Finish"}."Setup Parameters" ("Drive To Distance PID steps")) -> ()
                  n301 = global write "Robot Global Data.vi" "Drive To Distance Enable"(FALSE ("Drive To Distance Enable")) -> ()
                  n302 = global write "Robot Global Data.vi" "Autonomis States"(T10."End Auto" ("Autonomis States")) -> ()
                }
                frame "Place Gear Setup" {
                }
                frame "Place Gear Wait" {
                }
                frame "Place Gear End" {
                }
                frame "Angel Move Setup" {
                }
                frame "Angel Move Wait" {
                }
                frame "Angel Move End" {
                }
                frame "End Auto" {
                }
              }
            }
            frame True {
              n303 = global write "Robot Global Data.vi" "Autonomis init"(FALSE ("Autonomis init")) -> ()
              n304 = global write "Robot Global Data.vi" "Autonomis States"(T11."Move Distance Setup" ("Autonomis States")) -> ()
            }
          }
        }
      }
    }
    frame Enabled {
    }
  }
  n305 = disable-structure shown="Disabled" {
    frame Disabled {
      n306 = flat-sequence {
        frame #0 {
          n307 = global write "Robot Global Data.vi" "DriveYawControlComplete"(FALSE ("DriveYawControlRunning")) -> ()
          n308 = global write "Robot Global Data.vi" "Drive To Distance Complete"(FALSE ("Drive To Distance Complete")) -> ()
          n309 = global write "Robot Global Data.vi" "Drive Reset Encoders"(TRUE ("DriveYawControlRunning")) -> ()
          n310 = global write "Robot Global Data.vi" "Drive To Distance Enable"(FALSE ("Drive To Distance Enable")) -> ()
          n311 = global write "Robot Global Data.vi" "Drive to Angle"(FALSE ("Drive To Distance Enable")) -> ()
          n312 = global write "Robot Global Data.vi" "Drive To Distance PID steps"(enum16{"Setup Parameters", "Run PID", "Finish"}."Setup Parameters" ("Drive To Distance PID steps")) -> ()
          n313 = global write "Robot Global Data.vi" "Drive Striaght"(FALSE ("Drive To Distance Enable")) -> ()
          n314 = global write "Robot Global Data.vi" "Drive to Distance setpoint"(75.0 ("Drive to Distance setpoint")) -> ()
          n315 = global write "Robot Global Data.vi" "Nav Reset Yaw"(TRUE ("Drive To Distance Enable")) -> ()
          n316 = Wait (ms)(milliseconds to wait=u32 200) -> ()  [unwired: 1 out]
        }
        frame #1 {
          n317 = global write "Robot Global Data.vi" "Drive To Distance Enable"(TRUE ("Drive To Distance Enable")) -> ()
        }
        frame #2 {
          n318 = while {
            stop <- w303 stop-if-true
            n319 = global read "Robot Global Data.vi" "Drive To Distance Complete"() -> (w303:bool)
            n320 = Wait (ms)(milliseconds to wait=u32 10) -> ()  [unwired: 1 out]
          }
          n321 = global write "Robot Global Data.vi" "Drive Reset Encoders"(FALSE ("DriveYawControlRunning")) -> ()
        }
        frame #3 {
          n322 = global write "Robot Global Data.vi" "Drive To Distance Complete"(FALSE ("Drive To Distance Complete")) -> ()
          n323 = global write "Robot Global Data.vi" "DriveYawControlComplete"(FALSE ("DriveYawControlRunning")) -> ()
          n324 = global write "Robot Global Data.vi" "Drive to Angle"(TRUE ("Drive To Distance Enable")) -> ()
          n325 = global write "Robot Global Data.vi" "Drive Striaght"(FALSE ("Drive To Distance Enable")) -> ()
          n326 = global write "Robot Global Data.vi" "Drive Yaw Angle SP"(45.0 ("Drive Yaw Angle SP")) -> ()
          n327 = global write "Robot Global Data.vi" "Drive To Distance PID steps"(enum16{"Setup Parameters", "Run PID", "Finish"}."Setup Parameters" ("Drive To Distance PID steps")) -> ()
          n328 = global write "Robot Global Data.vi" "Drive To Distance Enable"(FALSE ("Drive To Distance Enable")) -> ()
        }
        frame #4 {
          n329 = while {
            stop <- w312 stop-if-true
            n330 = global read "Robot Global Data.vi" "DriveYawControlComplete"() -> (w312:bool)
            n331 = Wait (ms)(milliseconds to wait=u32 10) -> ()  [unwired: 1 out]
          }
        }
        frame #5 {
        }
        frame #6 {
          n332 = global write "Robot Global Data.vi" "DriveYawControlComplete"(FALSE ("DriveYawControlRunning")) -> ()
          n333 = global write "Robot Global Data.vi" "Drive To Distance Complete"(FALSE ("Drive To Distance Complete")) -> ()
          n334 = global write "Robot Global Data.vi" "Nav Reset Yaw"(FALSE ("Drive To Distance Enable")) -> ()
          n335 = global write "Robot Global Data.vi" "Drive to Distance setpoint"(36.0 ("Drive to Distance setpoint")) -> ()
          n336 = global write "Robot Global Data.vi" "Drive Reset Encoders"(TRUE ("DriveYawControlRunning")) -> ()
          n337 = global write "Robot Global Data.vi" "Drive To Distance PID steps"(enum16{"Setup Parameters", "Run PID", "Finish"}."Setup Parameters" ("Drive To Distance PID steps")) -> ()
          n338 = global write "Robot Global Data.vi" "Nav Reset Yaw"(FALSE ("Drive To Distance Enable")) -> ()
          n339 = global write "Robot Global Data.vi" "Drive to Angle"(FALSE ("Drive To Distance Enable")) -> ()
          n340 = global write "Robot Global Data.vi" "Drive Striaght"(FALSE ("Drive To Distance Enable")) -> ()
          n341 = Wait (ms)(milliseconds to wait=u32 50) -> ()  [unwired: 1 out]
        }
        frame #7 {
          n342 = global write "Robot Global Data.vi" "Drive To Distance Enable"(TRUE ("Drive To Distance Enable")) -> ()
        }
        frame #8 {
          n343 = while {
            stop <- w326 stop-if-true
            n344 = global read "Robot Global Data.vi" "Drive To Distance Complete"() -> (w326:bool)
            n345 = Wait (ms)(milliseconds to wait=u32 10) -> ()  [unwired: 1 out]
          }
          n346 = global write "Robot Global Data.vi" "Drive Reset Encoders"(FALSE ("DriveYawControlRunning")) -> ()
        }
        frame #9 {
          n347 = global write "Robot Global Data.vi" "DriveYawControlComplete"(FALSE ("DriveYawControlRunning")) -> ()
          n348 = global write "Robot Global Data.vi" "Drive To Distance Complete"(FALSE ("Drive To Distance Complete")) -> ()
          n349 = global write "Robot Global Data.vi" "Drive To Distance Enable"(FALSE ("Drive To Distance Enable")) -> ()
          n350 = global write "Robot Global Data.vi" "Drive Reset Encoders"(TRUE ("DriveYawControlRunning")) -> ()
          n351 = global write "Robot Global Data.vi" "Drive to Angle"(FALSE ("Drive To Distance Enable")) -> ()
          n352 = global write "Robot Global Data.vi" "Drive Striaght"(FALSE ("Drive To Distance Enable")) -> ()
        }
        frame #10 {
          n353 = global write "Robot Global Data.vi" "Drive Reset Encoders"(FALSE ("DriveYawControlRunning")) -> ()
        }
      }
    }
    frame Enabled {
    }
  }
  n354 = disable-structure shown="Disabled" {
    frame Disabled {
      n355 = flat-sequence {
        frame #0 {
          n356 = global write "Robot Global Data.vi" "DriveYawControlComplete"(FALSE ("DriveYawControlRunning")) -> ()
          n357 = global write "Robot Global Data.vi" "Drive To Distance Complete"(FALSE ("Drive To Distance Complete")) -> ()
          n358 = global write "Robot Global Data.vi" "Drive Reset Encoders"(TRUE ("DriveYawControlRunning")) -> ()
          n359 = global write "Robot Global Data.vi" "Drive To Distance Enable"(FALSE ("Drive To Distance Enable")) -> ()
          n360 = global write "Robot Global Data.vi" "Drive to Angle"(FALSE ("Drive To Distance Enable")) -> ()
          n361 = global write "Robot Global Data.vi" "Drive To Distance PID steps"(enum16{"Setup Parameters", "Run PID", "Finish"}."Setup Parameters" ("Drive To Distance PID steps")) -> ()
          n362 = global write "Robot Global Data.vi" "Drive Striaght"(FALSE ("Drive To Distance Enable")) -> ()
          n363 = global write "Robot Global Data.vi" "Drive to Distance setpoint"(75.0 ("Drive to Distance setpoint")) -> ()
          n364 = global write "Robot Global Data.vi" "Nav Reset Yaw"(TRUE ("Drive To Distance Enable")) -> ()
          n365 = Wait (ms)(milliseconds to wait=u32 200) -> ()  [unwired: 1 out]
        }
        frame #1 {
          n366 = global write "Robot Global Data.vi" "Drive To Distance Enable"(TRUE ("Drive To Distance Enable")) -> ()
        }
        frame #2 {
          n367 = while {
            stop <- w347 stop-if-true
            n368 = global read "Robot Global Data.vi" "Drive To Distance Complete"() -> (w347:bool)
            n369 = Wait (ms)(milliseconds to wait=u32 10) -> ()  [unwired: 1 out]
          }
          n370 = global write "Robot Global Data.vi" "Drive Reset Encoders"(FALSE ("DriveYawControlRunning")) -> ()
        }
        frame #3 {
          n371 = global write "Robot Global Data.vi" "Drive To Distance Complete"(FALSE ("Drive To Distance Complete")) -> ()
          n372 = global write "Robot Global Data.vi" "DriveYawControlComplete"(FALSE ("DriveYawControlRunning")) -> ()
          n373 = global write "Robot Global Data.vi" "Drive to Angle"(TRUE ("Drive To Distance Enable")) -> ()
          n374 = global write "Robot Global Data.vi" "Drive Striaght"(FALSE ("Drive To Distance Enable")) -> ()
          n375 = global write "Robot Global Data.vi" "Drive Yaw Angle SP"(45.0 ("Drive Yaw Angle SP")) -> ()
          n376 = global write "Robot Global Data.vi" "Drive To Distance PID steps"(enum16{"Setup Parameters", "Run PID", "Finish"}."Setup Parameters" ("Drive To Distance PID steps")) -> ()
          n377 = global write "Robot Global Data.vi" "Drive To Distance Enable"(FALSE ("Drive To Distance Enable")) -> ()
        }
        frame #4 {
          n378 = while {
            stop <- w356 stop-if-true
            n379 = global read "Robot Global Data.vi" "DriveYawControlComplete"() -> (w356:bool)
            n380 = Wait (ms)(milliseconds to wait=u32 10) -> ()  [unwired: 1 out]
          }
        }
        frame #5 {
        }
        frame #6 {
          n381 = global write "Robot Global Data.vi" "DriveYawControlComplete"(FALSE ("DriveYawControlRunning")) -> ()
          n382 = global write "Robot Global Data.vi" "Drive To Distance Complete"(FALSE ("Drive To Distance Complete")) -> ()
          n383 = global write "Robot Global Data.vi" "Nav Reset Yaw"(FALSE ("Drive To Distance Enable")) -> ()
          n384 = global write "Robot Global Data.vi" "Drive to Distance setpoint"(60.0 ("Drive to Distance setpoint")) -> ()
          n385 = global write "Robot Global Data.vi" "Drive Reset Encoders"(TRUE ("DriveYawControlRunning")) -> ()
          n386 = global write "Robot Global Data.vi" "Drive To Distance PID steps"(enum16{"Setup Parameters", "Run PID", "Finish"}."Setup Parameters" ("Drive To Distance PID steps")) -> ()
          n387 = global write "Robot Global Data.vi" "Nav Reset Yaw"(FALSE ("Drive To Distance Enable")) -> ()
          n388 = global write "Robot Global Data.vi" "Drive to Angle"(FALSE ("Drive To Distance Enable")) -> ()
          n389 = global write "Robot Global Data.vi" "Drive Striaght"(FALSE ("Drive To Distance Enable")) -> ()
          n390 = Wait (ms)(milliseconds to wait=u32 50) -> ()  [unwired: 1 out]
        }
        frame #7 {
          n391 = global write "Robot Global Data.vi" "Drive To Distance Enable"(TRUE ("Drive To Distance Enable")) -> ()
        }
        frame #8 {
          n392 = while {
            stop <- w370 stop-if-true
            n393 = global read "Robot Global Data.vi" "Drive To Distance Complete"() -> (w370:bool)
            n394 = Wait (ms)(milliseconds to wait=u32 10) -> ()  [unwired: 1 out]
          }
          n395 = global write "Robot Global Data.vi" "Drive Reset Encoders"(FALSE ("DriveYawControlRunning")) -> ()
        }
        frame #9 {
          n396 = global write "Robot Global Data.vi" "DriveYawControlComplete"(FALSE ("DriveYawControlRunning")) -> ()
          n397 = global write "Robot Global Data.vi" "Drive To Distance Complete"(FALSE ("Drive To Distance Complete")) -> ()
          n398 = global write "Robot Global Data.vi" "Drive To Distance Enable"(FALSE ("Drive To Distance Enable")) -> ()
          n399 = global write "Robot Global Data.vi" "Drive Reset Encoders"(TRUE ("DriveYawControlRunning")) -> ()
          n400 = global write "Robot Global Data.vi" "Drive to Angle"(FALSE ("Drive To Distance Enable")) -> ()
          n401 = global write "Robot Global Data.vi" "Drive Striaght"(FALSE ("Drive To Distance Enable")) -> ()
        }
        frame #10 {
          n402 = global write "Robot Global Data.vi" "Drive Reset Encoders"(FALSE ("DriveYawControlRunning")) -> ()
        }
      }
    }
    frame Enabled {
    }
  }
